vi "loadLSdata.vi"() -> ()   [LabVIEW 2012]
uses:
  <vilib>/Utility/file.llb/Read From Spreadsheet File (string).vi
  <vilib>/addons/database/Connection.llb/DB Tools Open Connec (Path).vi
  <vilib>/addons/database/NI_Database_API.lvlib
panel:
  out "error out 2":errorcluster
  out "error out":errorcluster
  out "element":i32
  out "Numeric":i32
  in  "Cluster":T1
  out "output cluster":T1
  out "first row":string[](array[string])
  in  "file path (dialog if empty)":path=path "C:/temp/LS/aa.csv"
  out "all rows":string[][](array[string])
  out "size(s)":i32[](array[numeric])
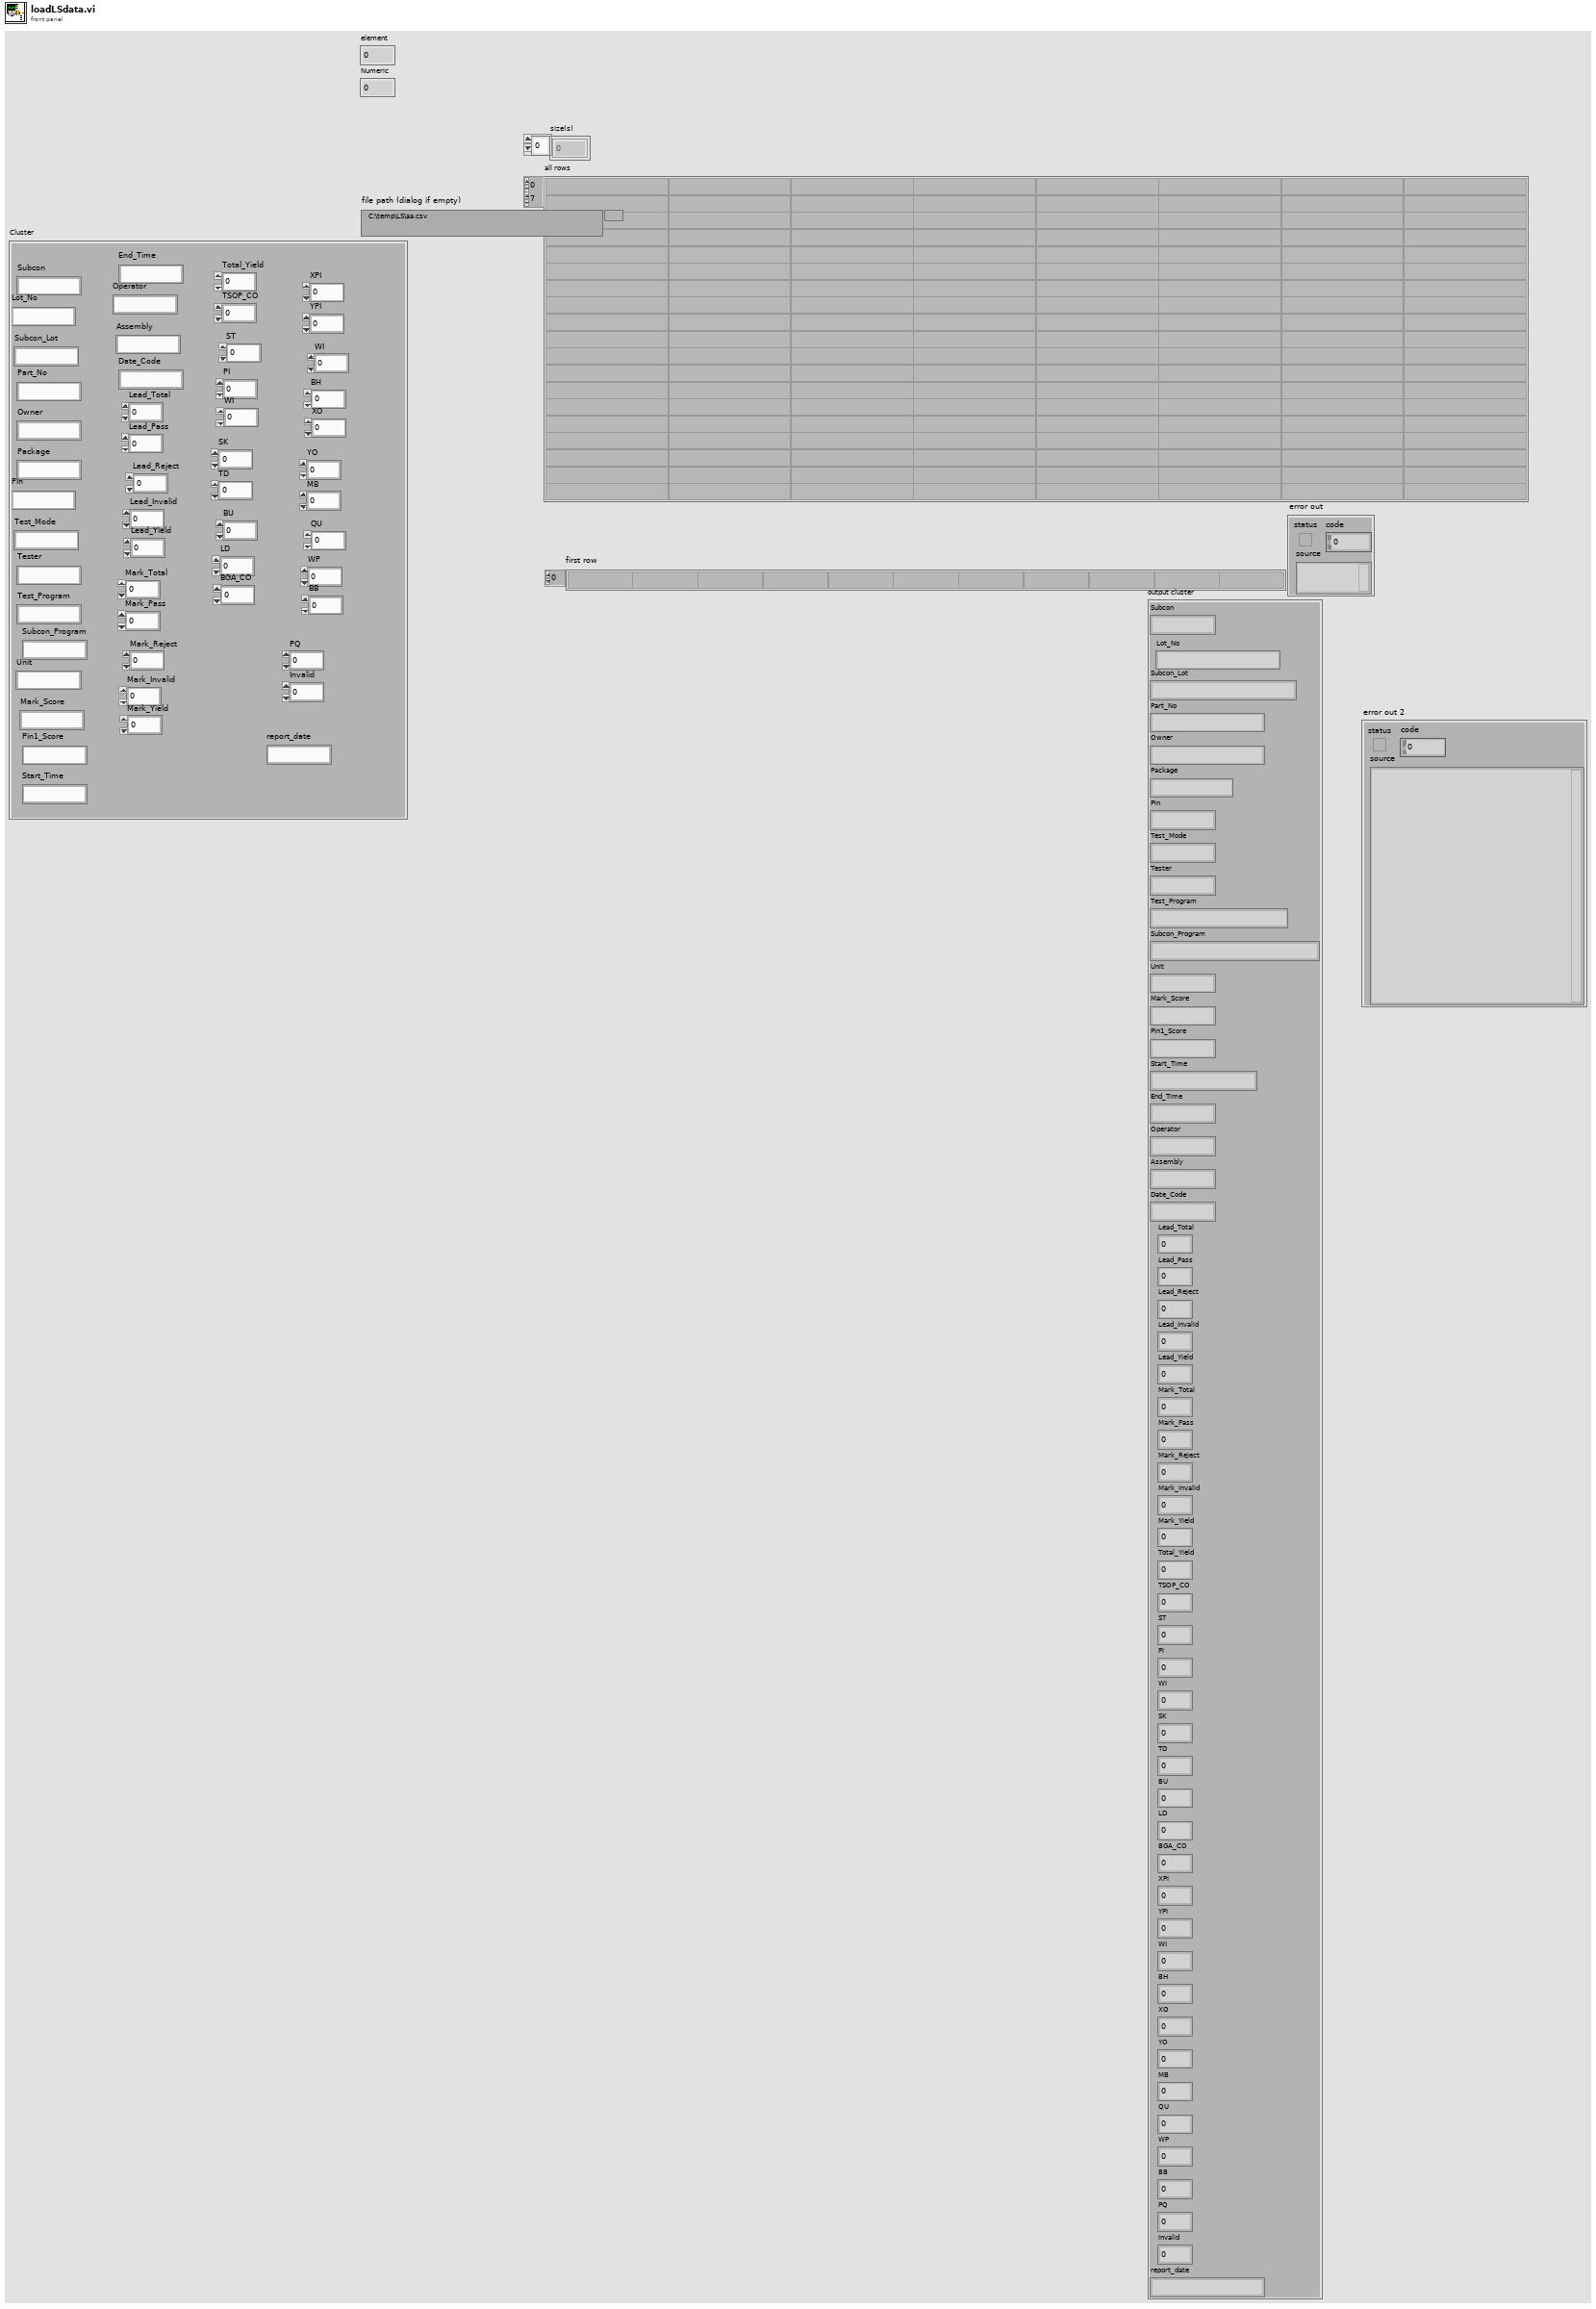
[diagram p1: front panel]
types:
  T1 = cluster{"Subcon":string, "Lot_No":string, "Subcon_Lot":string, "Part_No":string, "Owner":string, "Package":string, "Pin":string, "Test_Mode":string, "Tester":string, "Test_Program":string, "Subcon_Program":string, "Unit":string, "Mark_Score":string, "Pin1_Score":string, "Start_Time":string, "End_Time":string, "Operator":string, "Assembly":string, "Date_Code":string, "Lead_Total":dbl, "Lead_Pass":dbl, "Lead_Reject":dbl, "Lead_Invalid":dbl, "Lead_Yield":dbl, "Mark_Total":dbl, "Mark_Pass":dbl, "Mark_Reject":dbl, "Mark_Invalid":dbl, "Mark_Yield":dbl, "Total_Yield":dbl, "TSOP_CO":dbl, "ST":dbl, "PI":dbl, "WI":dbl, "SK":dbl, "TD":dbl, "BU":dbl, "LD":dbl, "BGA_CO":dbl, "XPI":dbl, "YPI":dbl, "WI":dbl, "BH":dbl, "XO":dbl, "YO":dbl, "MB":dbl, "QU":dbl, "WP":dbl, "BB":dbl, "PQ":dbl, "Invalid":dbl, "report_date":string}
  T2 = typedef "NI_Database_API.lvlib/Conn ObjectReference.ctl" = refnum<k1>
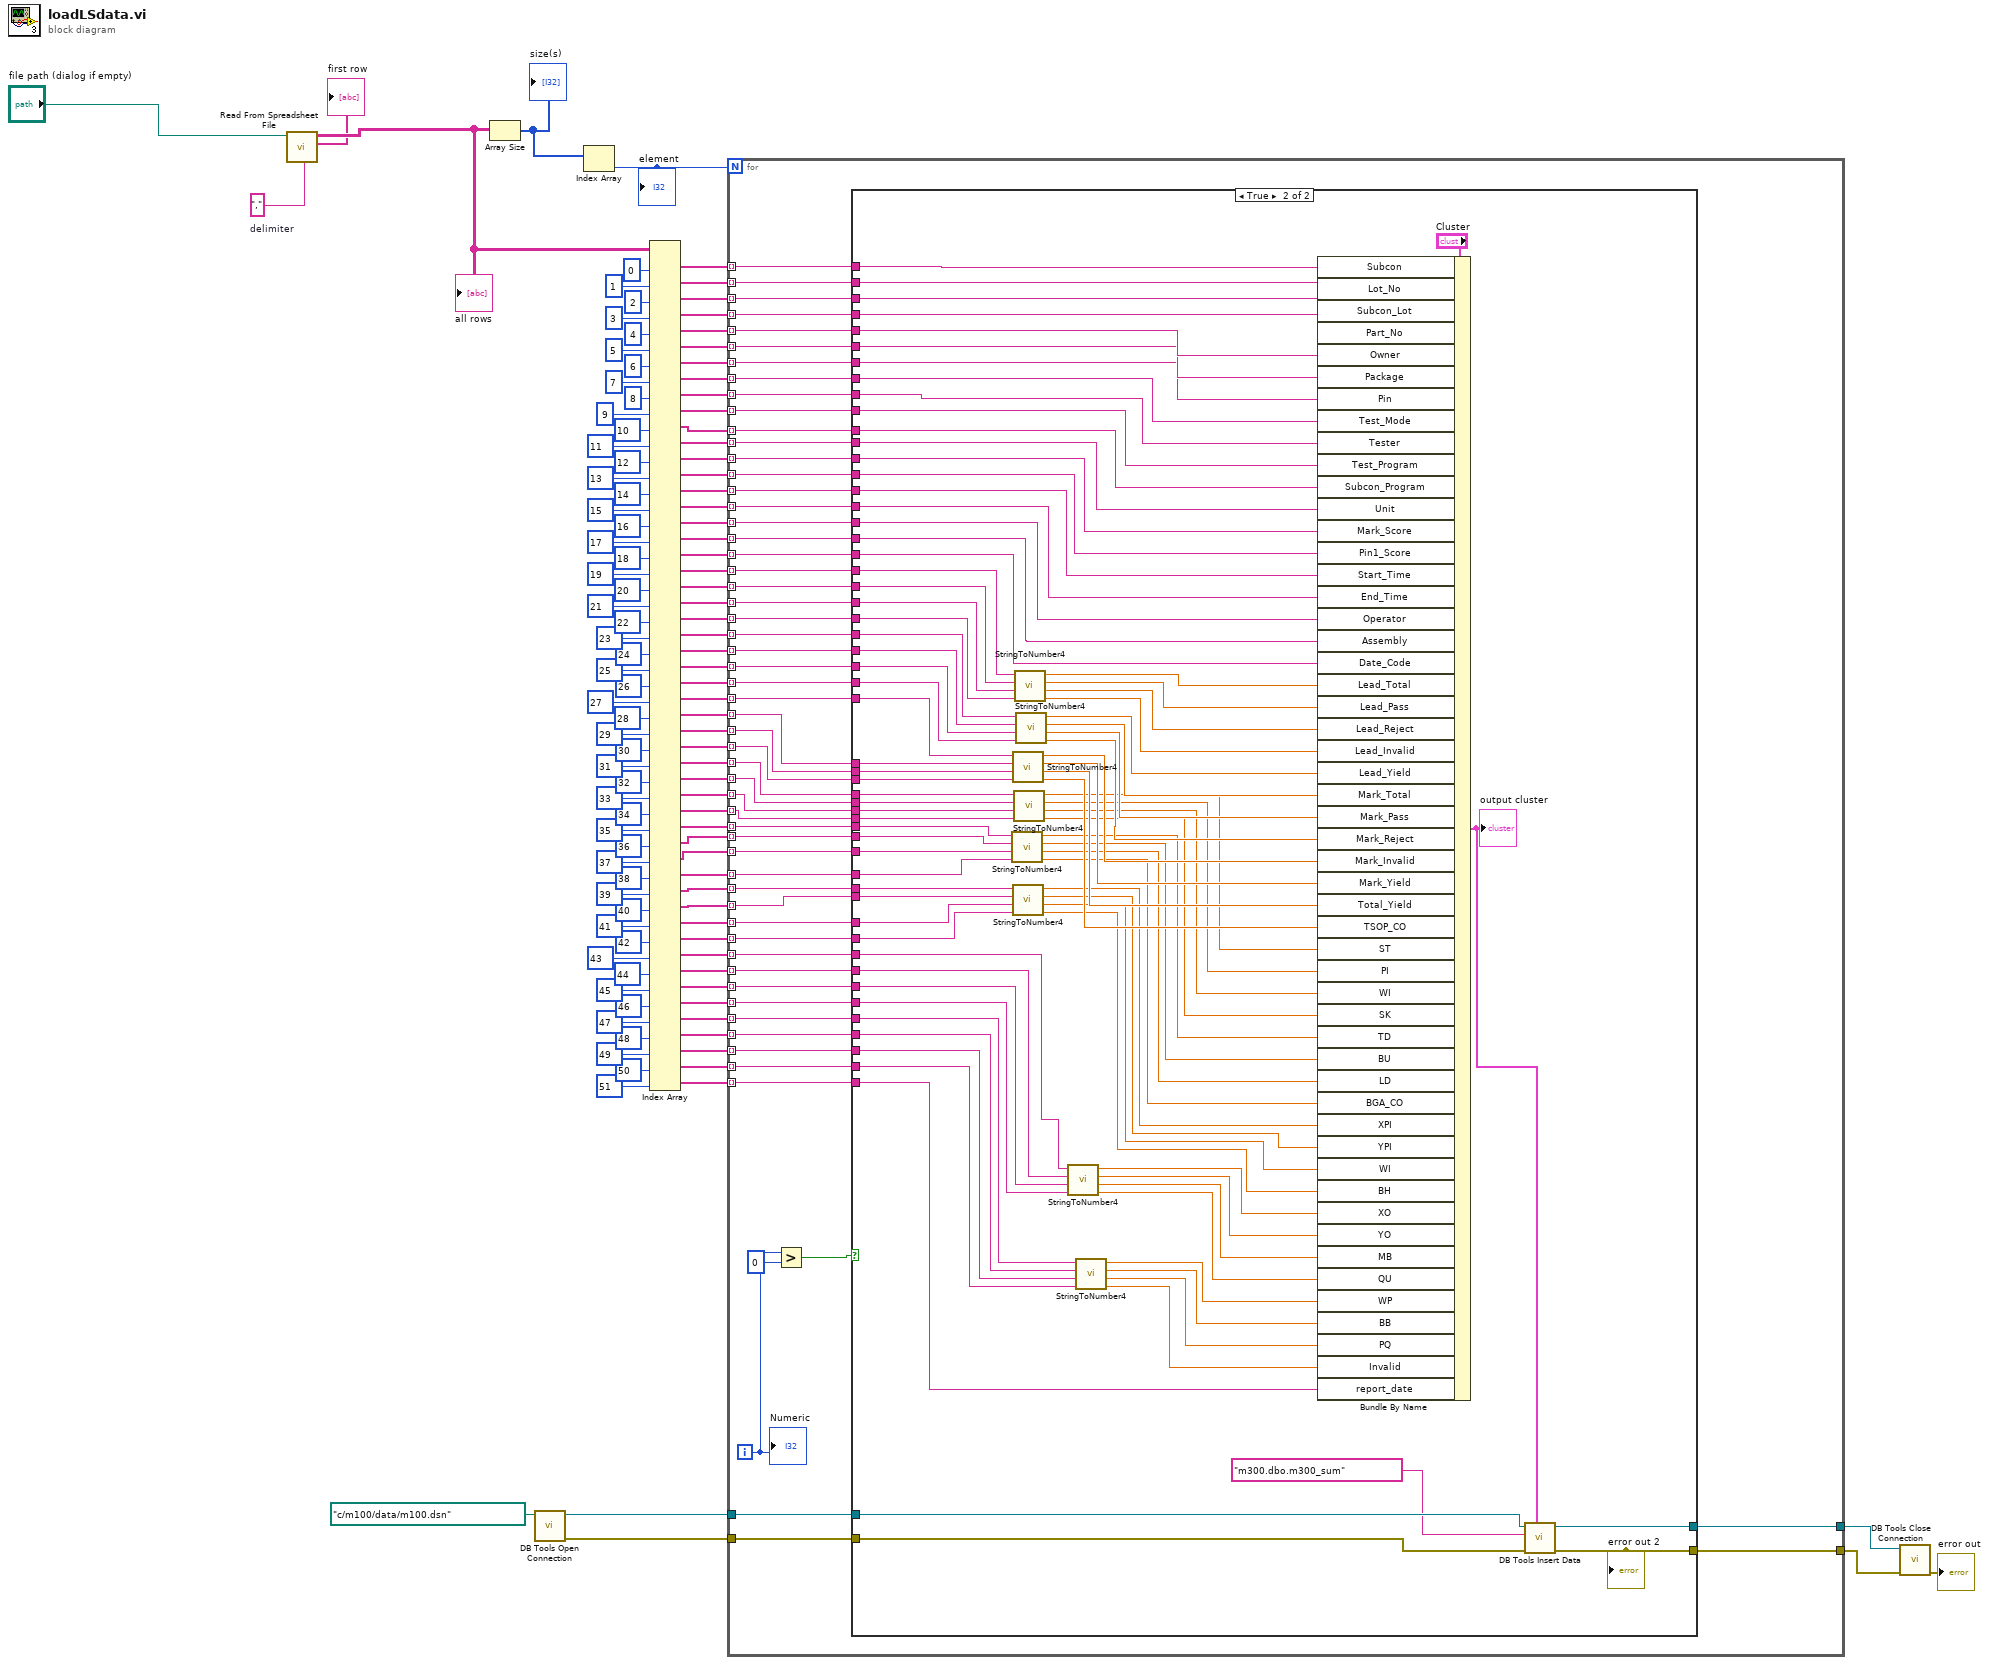
[diagram p0: block diagram]
diagram:
  w116 = ","  # delimiter
  n1 = call-poly <vilib>:"Read From Spreadsheet File.vi"("delimiter (\\t)"=w116, "file path (dialog if empty)"="file path (dialog if empty)") -> ("first row"=→"first row":string[], "all rows"=w115:string[][])  [unwired: 5 in, 3 out]
  "all rows" <- w115
  n2 = Array Size(array=w115) -> (size(s)=w8:i32[])
  "size(s)" <- w8
  n3 = call-poly <vilib>:"DB Tools Open Connection.vi"("connection information"=path "c:/m100/data/m100.dsn") -> ("error out"=w4:errorcluster, "connection reference"=w5:T2)  [unwired: 7 in]
  n4 = Index Array(array=w8) -> (element=w7:i32)  [unwired: 1 in]
  "element" <- w7
  n5 = Index Array(array=w115, index (col) #1=0 ("disabled index (col)"), index (col) #2=1 ("index (col)"), index (col) #3=2 ("index (col)"), index (col) #4=3 ("index (col)"), index (col) #5=4 ("index (col)"), index (col) #6=5 ("index (col)"), index (col) #7=6 ("index (col)"), index (col) #8=7 ("index (col)"), index (col) #9=8 ("index (col)"), index (col) #10=9 ("index (col)"), index (col) #11=10 ("index (col)"), index (col) #12=11 ("index (col)"), index (col) #13=12 ("index (col)"), index (col) #14=13 ("index (col)"), index (col) #15=14 ("index (col)"), index (col) #16=15 ("index (col)"), index (col) #17=16 ("index (col)"), index (col) #18=17 ("index (col)"), index (col) #19=18 ("index (col)"), index (col) #20=19 ("index (col)"), index (col) #21=20 ("index (col)"), index (col) #22=21 ("index (col)"), index (col) #23=22 ("index (col)"), index (col) #24=23 ("index (col)"), index (col) #25=24 ("index (col)"), index (col) #26=25 ("index (col)"), index (col) #27=26 ("index (col)"), index (col) #28=27 ("index (col)"), index (col) #29=28 ("index (col)"), index (col) #30=29 ("index (col)"), index (col) #31=30 ("index (col)"), index (col) #32=31 ("index (col)"), index (col) #33=32 ("index (col)"), index (col) #34=33 ("index (col)"), index (col) #35=34 ("index (col)"), index (col) #36=35 ("index (col)"), index (col) #37=36 ("index (col)"), index (col) #38=37 ("index (col)"), index (col) #39=38 ("index (col)"), index (col) #40=39 ("index (col)"), index (col) #41=40 ("index (col)"), index (col) #42=41 ("index (col)"), index (col) #43=42 ("index (col)"), index (col) #44=43 ("index (col)"), index (col) #45=44 ("index (col)"), index (col) #46=45 ("index (col)"), index (col) #47=46 ("index (col)"), index (col) #48=47 ("index (col)"), index (col) #49=48 ("index (col)"), index (col) #50=49 ("index (col)"), index (col) #51=50 ("index (col)"), index (col) #52=51 ("index (col)")) -> (element #1=w90:string[], element #2=w89:string[], element #3=w88:string[], element #4=w87:string[], element #5=w86:string[], element #6=w85:string[], element #7=w84:string[], element #8=w83:string[], element #9=w82:string[], element #10=w81:string[], element #11=w80:string[], element #12=w79:string[], element #13=w78:string[], element #14=w77:string[], element #15=w76:string[], element #16=w75:string[], element #17=w74:string[], element #18=w73:string[], element #19=w72:string[], element #20=w71:string[], element #21=w58:string[], element #22=w57:string[], element #23=w56:string[], element #24=w55:string[], element #25=w54:string[], element #26=w53:string[], element #27=w52:string[], element #28=w51:string[], element #29=w50:string[], element #30=w49:string[], element #31=w48:string[], element #32=w47:string[], element #33=w46:string[], element #34=w45:string[], element #35=w44:string[], element #36=w43:string[], element #37=w42:string[], element #38=w41:string[], element #39=w40:string[], element #40=w39:string[], element #41=w38:string[], element #42=w37:string[], element #43=w36:string[], element #44=w26:string[], element #45=w25:string[], element #46=w24:string[], element #47=w23:string[], element #48=w22:string[], element #49=w21:string[], element #50=w20:string[], element #51=w19:string[], element #52=w18:string[])  [unwired: 52 in]
  n6 = for {
    N: w7 -> [_]
    tunnel: w90 -> [w175] mode=indexing
    tunnel: w89 -> [w174] mode=indexing
    tunnel: w88 -> [w173] mode=indexing
    tunnel: w87 -> [w172] mode=indexing
    tunnel: w86 -> [w171] mode=indexing
    tunnel: w85 -> [w170] mode=indexing
    tunnel: w84 -> [w169] mode=indexing
    tunnel: w83 -> [w168] mode=indexing
    tunnel: w82 -> [w167] mode=indexing
    tunnel: w81 -> [w166] mode=indexing
    tunnel: w80 -> [w165] mode=indexing
    tunnel: w79 -> [w164] mode=indexing
    tunnel: w78 -> [w163] mode=indexing
    tunnel: w77 -> [w162] mode=indexing
    tunnel: w76 -> [w161] mode=indexing
    tunnel: w75 -> [w160] mode=indexing
    tunnel: w74 -> [w159] mode=indexing
    tunnel: w73 -> [w158] mode=indexing
    tunnel: w72 -> [w157] mode=indexing
    tunnel: w71 -> [w156] mode=indexing
    tunnel: w58 -> [w155] mode=indexing
    tunnel: w57 -> [w154] mode=indexing
    tunnel: w56 -> [w153] mode=indexing
    tunnel: w55 -> [w152] mode=indexing
    tunnel: w54 -> [w151] mode=indexing
    tunnel: w53 -> [w150] mode=indexing
    tunnel: w52 -> [w149] mode=indexing
    tunnel: w51 -> [w148] mode=indexing
    tunnel: w50 -> [w147] mode=indexing
    tunnel: w49 -> [w146] mode=indexing
    tunnel: w48 -> [w145] mode=indexing
    tunnel: w47 -> [w144] mode=indexing
    tunnel: w46 -> [w143] mode=indexing
    tunnel: w45 -> [w142] mode=indexing
    tunnel: w44 -> [w141] mode=indexing
    tunnel: w43 -> [w140] mode=indexing
    tunnel: w42 -> [w139] mode=indexing
    tunnel: w41 -> [w138] mode=indexing
    tunnel: w40 -> [w137] mode=indexing
    tunnel: w39 -> [w136] mode=indexing
    tunnel: w38 -> [w135] mode=indexing
    tunnel: w37 -> [w134] mode=indexing
    tunnel: w36 -> [w133] mode=indexing
    tunnel: w26 -> [w132] mode=indexing
    tunnel: w25 -> [w131] mode=indexing
    tunnel: w24 -> [w130] mode=indexing
    tunnel: w23 -> [w129] mode=indexing
    tunnel: w22 -> [w128] mode=indexing
    tunnel: w21 -> [w127] mode=indexing
    tunnel: w20 -> [w126] mode=indexing
    tunnel: w19 -> [w125] mode=indexing
    tunnel: w18 -> [w124] mode=indexing
    tunnel: w5 -> [w120]
    tunnel: w4 -> [w119]
    tunnel: [w118] -> w3
    tunnel: [w117] -> w2
    i -> [w123]
    n7 = Greater?(x=w123, y=0) -> (0:w121:bool)
    n8 = case shown="True" w121 {
      tunnel: w175 -> [_ w267]
      tunnel: w174 -> [_ w266]
      tunnel: w173 -> [_ w265]
      tunnel: w172 -> [_ w264]
      tunnel: w171 -> [_ w263]
      tunnel: w170 -> [_ w262]
      tunnel: w169 -> [_ w261]
      tunnel: w168 -> [_ w260]
      tunnel: w167 -> [_ w259]
      tunnel: w166 -> [_ w258]
      tunnel: w165 -> [_ w257]
      tunnel: w164 -> [_ w256]
      tunnel: w163 -> [_ w255]
      tunnel: w162 -> [_ w254]
      tunnel: w161 -> [_ w253]
      tunnel: w160 -> [_ w252]
      tunnel: w159 -> [_ w251]
      tunnel: w158 -> [_ w250]
      tunnel: w157 -> [_ w249]
      tunnel: w156 -> [_ w248]
      tunnel: w155 -> [_ w247]
      tunnel: w154 -> [_ w246]
      tunnel: w153 -> [_ w245]
      tunnel: w152 -> [_ w244]
      tunnel: w151 -> [_ w243]
      tunnel: w150 -> [_ w242]
      tunnel: w149 -> [_ w241]
      tunnel: w148 -> [_ w240]
      tunnel: w147 -> [_ w239]
      tunnel: w146 -> [_ w238]
      tunnel: w145 -> [_ w237]
      tunnel: w144 -> [_ w224]
      tunnel: w143 -> [_ w223]
      tunnel: w142 -> [_ w222]
      tunnel: w141 -> [_ w221]
      tunnel: w140 -> [_ w220]
      tunnel: w139 -> [_ w219]
      tunnel: w138 -> [_ w218]
      tunnel: w137 -> [_ w217]
      tunnel: w136 -> [_ w216]
      tunnel: w135 -> [_ w215]
      tunnel: w134 -> [_ w214]
      tunnel: w133 -> [_ w213]
      tunnel: w132 -> [_ w212]
      tunnel: w131 -> [_ w211]
      tunnel: w130 -> [_ w210]
      tunnel: w129 -> [_ w209]
      tunnel: w128 -> [_ w208]
      tunnel: w127 -> [_ w207]
      tunnel: w126 -> [_ w206]
      tunnel: w125 -> [_ w205]
      tunnel: w124 -> [_ w204]
      tunnel: w120 -> [w177 w183]
      tunnel: w119 -> [w176 w182]
      tunnel: [w177 w179] -> w118
      tunnel: [w176 w178] -> w117
      frame False {
      }
      frame True {
        n9 = call "StringToNumber4.vi"("string 4"=w217, "string 3"=w218, "string 2"=w219, "string"=w220) -> ("Numeric 4"=w196:dbl, "Numeric 3"=w197:dbl, "Numeric 2"=w198:dbl, "Numeric"=w199:dbl)  [unwired: 4 in]
        n10 = call "StringToNumber4.vi"("string 4"=w237, "string 3"=w238, "string 2"=w239, "string"=w240) -> ("Numeric 4"=w225:dbl, "Numeric 3"=w226:dbl, "Numeric 2"=w227:dbl, "Numeric"=w228:dbl)  [unwired: 4 in]
        n11 = call "StringToNumber4.vi"("string 4"=w213, "string 3"=w214, "string 2"=w215, "string"=w216) -> ("Numeric 4"=w192:dbl, "Numeric 3"=w193:dbl, "Numeric 2"=w194:dbl, "Numeric"=w195:dbl)  [unwired: 4 in]
        n12 = call "StringToNumber4.vi"("string 4"=w221, "string 3"=w222, "string 2"=w223, "string"=w224) -> ("Numeric 4"=w200:dbl, "Numeric 3"=w201:dbl, "Numeric 2"=w202:dbl, "Numeric"=w203:dbl)  [unwired: 4 in]
        n13 = call "StringToNumber4.vi"("string 4"=w245, "string 3"=w246, "string 2"=w247, "string"=w248) -> ("Numeric 4"=w233:dbl, "Numeric 3"=w234:dbl, "Numeric 2"=w235:dbl, "Numeric"=w236:dbl)  [unwired: 4 in]
        n14 = call "StringToNumber4.vi"("string 4"=w241, "string 3"=w242, "string 2"=w243, "string"=w244) -> ("Numeric 4"=w229:dbl, "Numeric 3"=w230:dbl, "Numeric 2"=w231:dbl, "Numeric"=w232:dbl)  [unwired: 4 in]
        n15 = call "StringToNumber4.vi"("string 4"=w209, "string 3"=w210, "string 2"=w211, "string"=w212) -> ("Numeric 4"=w188:dbl, "Numeric 3"=w189:dbl, "Numeric 2"=w190:dbl, "Numeric"=w191:dbl)  [unwired: 4 in]
        n16 = call "StringToNumber4.vi"("string 4"=w205, "string 3"=w206, "string 2"=w207, "string"=w208) -> ("Numeric 4"=w184:dbl, "Numeric 3"=w185:dbl, "Numeric 2"=w186:dbl, "Numeric"=w187:dbl)  [unwired: 4 in]
        n17 = Bundle By Name(cluster="Cluster", "Subcon"=w267, "Lot_No"=w266, "Subcon_Lot"=w265, "Part_No"=w264, "Owner"=w263, "Package"=w262, "Pin"=w261, "Test_Mode"=w260, "Tester"=w259, "Test_Program"=w258, "Subcon_Program"=w257, "Unit"=w256, "Mark_Score"=w255, "Pin1_Score"=w254, "Start_Time"=w253, "End_Time"=w252, "Operator"=w251, "Assembly"=w250, "Date_Code"=w249, "Lead_Total"=w236, "Lead_Pass"=w235, "Lead_Reject"=w234, "Lead_Invalid"=w233, "Lead_Yield"=w232, "Mark_Total"=w231, "Mark_Pass"=w230, "Mark_Reject"=w229, "Mark_Invalid"=w228, "Mark_Yield"=w227, "Total_Yield"=w226, "TSOP_CO"=w225, "ST"=w203, "PI"=w202, "WI"=w201, "SK"=w200, "TD"=w199, "BU"=w198, "LD"=w197, "BGA_CO"=w196, "XPI"=w195, "YPI"=w194, "WI"=w193, "BH"=w192, "XO"=w191, "YO"=w190, "MB"=w189, "QU"=w188, "WP"=w187, "BB"=w186, "PQ"=w185, "Invalid"=w184, "report_date"=w204) -> (w180:T1)
        "output cluster" <- w180
        n18 = call <vilib>:"DB Tools Insert Data.vi"("data"=w180, "error in (no error)"=w182, "table"="m300.dbo.m300_sum", "connection reference"=w183) -> ("error out"=w178:errorcluster, "connection reference out"=w179:T2)  [unwired: 6 in]
        "error out 2" <- w178
      }
    }
    "Numeric" <- w123
  }
  n19 = call <vilib>:"DB Tools Close Connection.vi"("error in (no error)"=w2, "connection reference"=w3) -> ("error out"=→"error out":errorcluster)  [unwired: 5 in]
